vi "CreateTestSuite.vi"(5 "TestSuite In":refnum<class "TestSuite.lvclass">, 8 "error in (no error)":errorcluster, 11 "Name":string) -> (0 "error out":errorcluster, 3 "TestSuite":refnum<class "TestSuite.lvclass">)   [LabVIEW 2019, in "TestSuite.lvclass"]
uses:
  TestSuite.lvclass
  TestSuite.lvclass/TestSuite.ctl
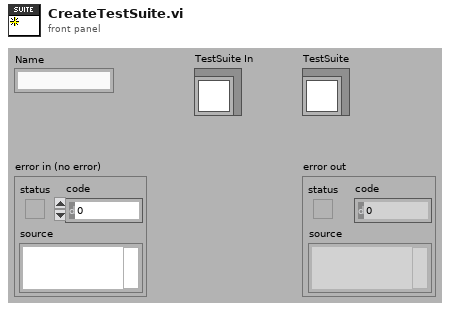
[diagram p1: front panel]
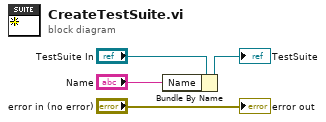
[diagram p0: block diagram]
diagram:
  n1 = Bundle By Name(cluster="TestSuite In", "Name"="Name") -> (→"TestSuite":refnum<class "TestSuite.lvclass">)
  "error out" <- "error in (no error)"
